vi "流程汇总.vi"(6 "CODMn量程切换":enum32{"H", "L", "AUTO"}(ring)=enum."AUTO", 8 "总磷量程切换":enum32{"H", "L", "AUTO"}(ring)=enum."AUTO", 9 "总氮量程切换":enum32{"H", "L", "AUTO"}(ring)=enum."AUTO", 10 "氨氮量程切换":enum32{"H", "L", "AUTO"}(ring)=enum."AUTO", 11 "参数":T1={"是否启用仪器"=FALSE, "CODMn"={"启动测量模式"={"测量模式"=enum."水样测量"}, "确定按钮"=TRUE}, "启动模块"={"氨氮"=FALSE, "总磷"=FALSE, "总氮"=FALSE, "CODMn"=FALSE, "CODCr"=FALSE}, "常规启动"=FALSE, "直接启动"=FALSE}) -> ()   [LabVIEW 2016]
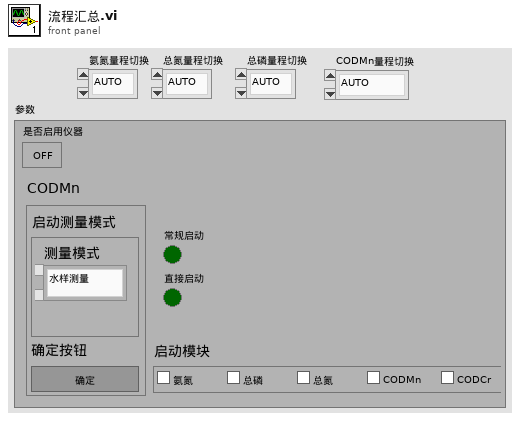
[diagram p1: front panel]
types:
  T1 = cluster{"是否启用仪器":bool, "CODMn":cluster{"启动测量模式":cluster{"测量模式":enum16{"水样测量", "标样核查", "加标回收", "平行样", "校零", "校标"}}, "确定按钮":bool}, "启动模块":cluster{"氨氮":bool, "总磷":bool, "总氮":bool, "CODMn":bool, "CODCr":bool}, "常规启动":bool, "直接启动":bool}
  T2 = enum32{"Bad", "Idle", "Run top level", "Running"}
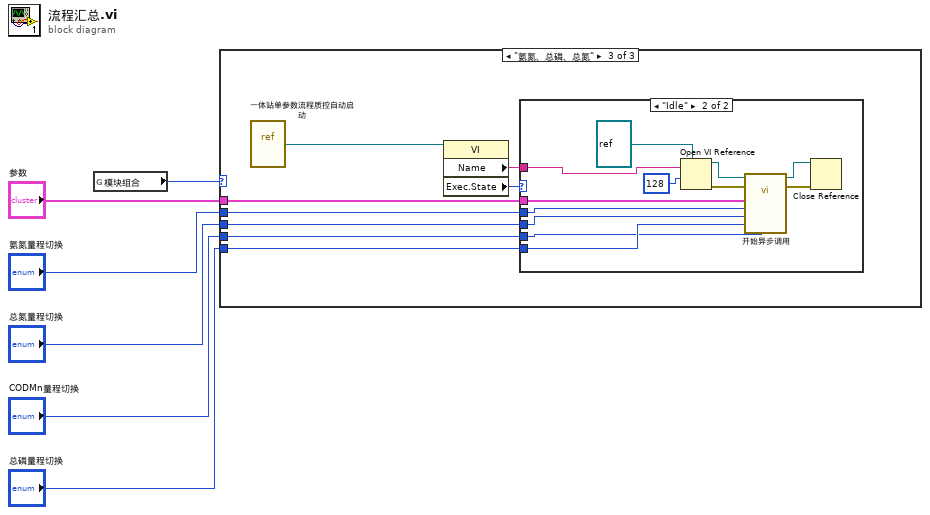
[diagram p0: block diagram]
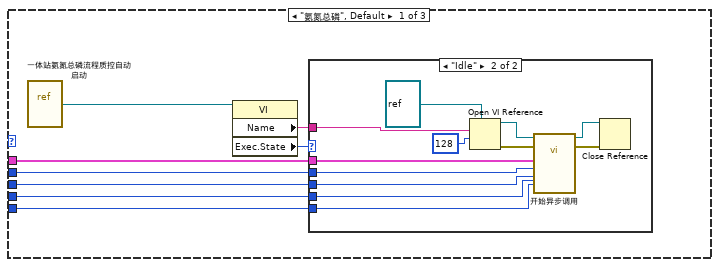
[diagram p2: hidden frame]
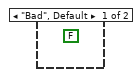
[diagram p3: hidden frame]
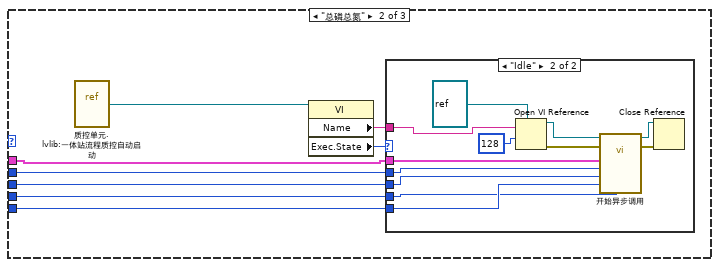
[diagram p4: hidden frame]
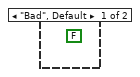
[diagram p5: hidden frame]
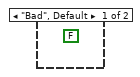
[diagram p6: hidden frame]
diagram:
  n1 = global read "断电保存全局.vi" "模块组合"() -> (w6:enum16{"氨氮总磷", "总磷总氮", "氨氮、总磷、总氮"})
  n2 = case shown="\"氨氮、总磷、总氮\"" w6 {
    tunnel: "参数" -> [w11 w31 w51]
    tunnel: "氨氮量程切换" -> [w10 w30 w50]
    tunnel: "总氮量程切换" -> [w9 w29 w49]
    tunnel: "总磷量程切换" -> [w8 w28 w48]
    tunnel: "CODMn量程切换" -> [w7 w27 w47]
    frame "氨氮总磷", Default {
      n3 = vi-ref "一体站氨氮总磷流程质控自动启动.vi"() -> (w14:refnum<vi>)
      n4 = property class="VI"(reference=w14) -> ("Name"=w12:string, "Exec.State"=w13:T2)  [unwired: 1 in, 2 out]
      n5 = case shown="\"Idle\"" w13 {
        tunnel: w12 -> [_ w26]
        tunnel: w11 -> [_ w19]
        tunnel: w10 -> [_ w18]
        tunnel: w9 -> [_ w17]
        tunnel: w8 -> [_ w16]
        tunnel: w7 -> [_ w15]
        frame "Bad", Default {
          (unwired) FALSE
        }
        frame "Idle" {
          n6 = Open VI Reference(type specifier VI Refnum (for type only)=refnum<vi> refnum ("类型说明符VI引用句柄（仅用于类型）"), vi path=w26, options=128 ("选项")) -> (vi reference=w25:refnum<vi>, error out=w22:errorcluster)  [unwired: 3 in]
          n7 = call-by-ref "开始异步调用"(reference=w25, error in=w22, "CODMn量程切换"=w15, "总磷量程切换"=w16, "总氮量程切换"=w17, "氨氮量程切换"=w18, "参数"=w19) -> (reference out=w24:refnum<vi>, error out=w23:errorcluster)  [unwired: 7 in]
          n8 = Close Reference(reference=w24, error in (no error)=w23) -> ()  [unwired: 1 out]
        }
      }
    }
    frame "总磷总氮" {
      n9 = vi-ref "质控单元.lvlib:一体站流程质控自动启动.vi"() -> (w34:refnum<vi>)
      n10 = property class="VI"(reference=w34) -> ("Name"=w32:string, "Exec.State"=w33:T2)  [unwired: 1 in, 2 out]
      n11 = case shown="\"Idle\"" w33 {
        tunnel: w32 -> [_ w46]
        tunnel: w31 -> [_ w39]
        tunnel: w30 -> [_ w38]
        tunnel: w29 -> [_ w37]
        tunnel: w28 -> [_ w36]
        tunnel: w27 -> [_ w35]
        frame "Bad", Default {
          (unwired) FALSE
        }
        frame "Idle" {
          n12 = Open VI Reference(type specifier VI Refnum (for type only)=refnum<vi> refnum ("类型说明符VI引用句柄（仅用于类型）"), vi path=w46, options=128 ("选项")) -> (vi reference=w45:refnum<vi>, error out=w42:errorcluster)  [unwired: 3 in]
          n13 = call-by-ref "开始异步调用"(reference=w45, error in=w42, "CODMn量程切换"=w35, "总磷量程切换"=w36, "总氮量程切换"=w37, "氨氮量程切换"=w38, "参数"=w39) -> (reference out=w44:refnum<vi>, error out=w43:errorcluster)  [unwired: 7 in]
          n14 = Close Reference(reference=w44, error in (no error)=w43) -> ()  [unwired: 1 out]
        }
      }
    }
    frame "氨氮、总磷、总氮" {
      n15 = vi-ref "一体站单参数流程质控自动启动.vi"() -> (w54:refnum<vi>)
      n16 = property class="VI"(reference=w54) -> ("Name"=w52:string, "Exec.State"=w53:T2)  [unwired: 1 in, 2 out]
      n17 = case shown="\"Idle\"" w53 {
        tunnel: w52 -> [_ w66]
        tunnel: w51 -> [_ w59]
        tunnel: w50 -> [_ w58]
        tunnel: w49 -> [_ w57]
        tunnel: w48 -> [_ w56]
        tunnel: w47 -> [_ w55]
        frame "Bad", Default {
          (unwired) FALSE
        }
        frame "Idle" {
          n18 = Open VI Reference(type specifier VI Refnum (for type only)=refnum<vi> refnum ("类型说明符VI引用句柄（仅用于类型）"), vi path=w66, options=128 ("选项")) -> (vi reference=w65:refnum<vi>, error out=w62:errorcluster)  [unwired: 3 in]
          n19 = call-by-ref "开始异步调用"(reference=w65, error in=w62, "CODMn量程切换"=w55, "总磷量程切换"=w56, "总氮量程切换"=w57, "氨氮量程切换"=w58, "参数"=w59) -> (reference out=w64:refnum<vi>, error out=w63:errorcluster)  [unwired: 7 in]
          n20 = Close Reference(reference=w64, error in (no error)=w63) -> ()  [unwired: 1 out]
        }
      }
    }
  }
